vi "Tom_Bentham_Flux.vi"() -> (5 "Plug in titles":string[](array[string]), 7 "Plug in values":string[](array[string]))   [LabVIEW 2010]
uses:
  Globals/Plug_in_data_global.vi
  Globals/Meas_global.vi
  Globals/LDA_meas_global_1.vi
panel:
  in  "FFID  Channel":u16(ring)=2 items=["LDA (U)", "LDA (W)", "FF (C) Sync", "FF (C)"]
  in  "Flux velocity Channel":u16(ring) items=["LDA (U)", "LDA (W)", "FF (C) Sync", "FF (C)"]
  out "Flux":cluster{"Histogram of X":dbl[], "Axis":dbl[]}(graph)
  out "FF":cluster{"Histogram of X":dbl[], "Axis":dbl[]}(graph)
  out "LDA 1st Comp":cluster{"Histogram of X":dbl[], "Axis":dbl[]}(graph)
  out "LDA 2nd Comp":cluster{"Histogram of X":dbl[], "Axis":dbl[]}(graph)
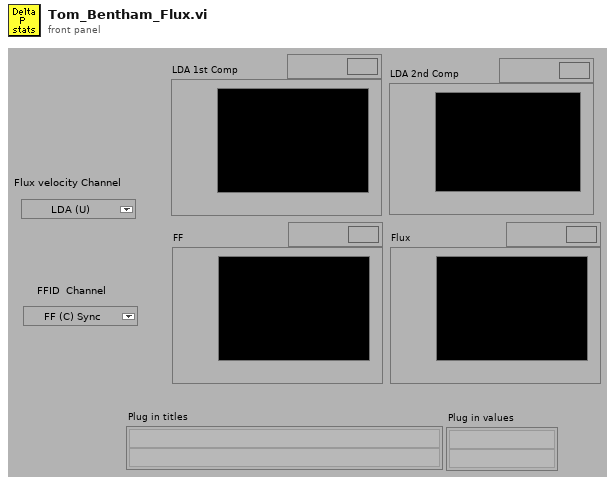
[diagram p1: front panel]
types:
  T1 = typedef "Analysis_info_cluster.ctl" = cluster{"Colour":u32, "Inst type":T2, "Inst name":string, "Symbol":string, "Code name":string, "Extra Info":string, "Inst Array":T3, "Index":i32, "Voltage Index":i32, "Extra Titles":string[], "Extra Values":string[]}
  T2 = typedef "Inst_type.ctl" = enum16{"Propeller anemometer", "Raw voltage", "Pressure Transducer", "Pitot-static tube", "Preston tube", "Hot wire", "Cross wire 1", "Cross wire 2", "Generic Linear", "Generic Polynomial", "Generic BackPoly", "Fast FID", "Thermocouple", "Cold wire", "Pulsed Wire", "LDA Vel", "LDA Tran time", "LDA Arr time"}
  T3 = typedef "Instrument_Array.ctl" = enum16{"PWA", "LDA", "Analogue"}
  T4 = enum16{"Save no data", "Save data in new files", "Save data in existing files"}
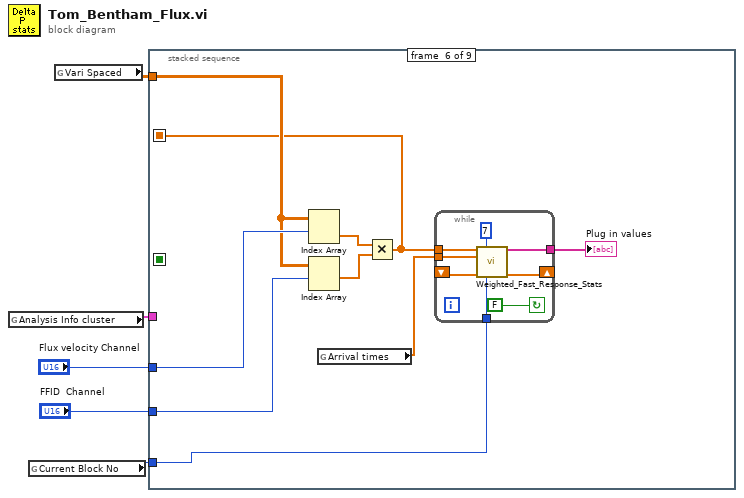
[diagram p0: block diagram]
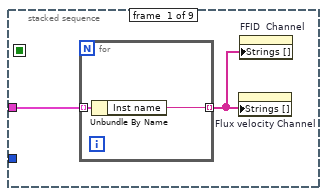
[diagram p2: hidden frame]
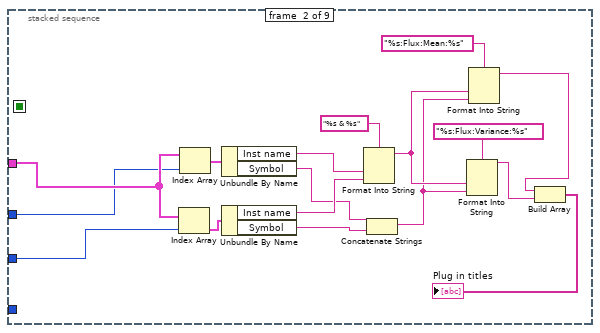
[diagram p3: hidden frame]
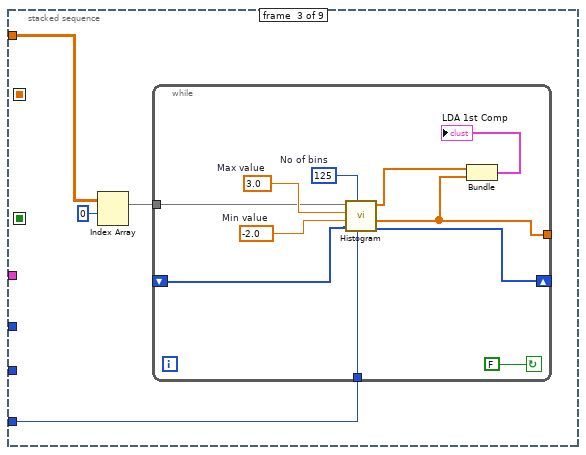
[diagram p4: hidden frame]
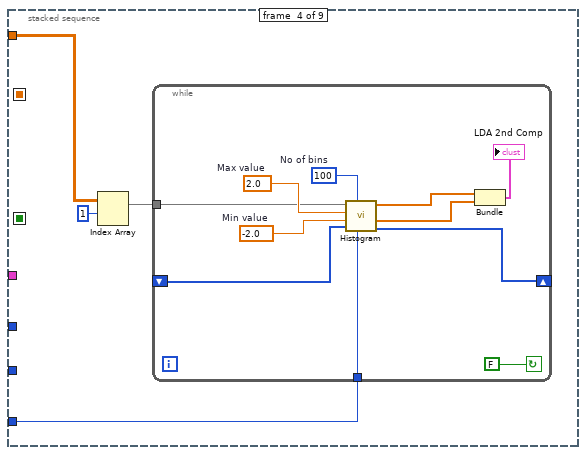
[diagram p5: hidden frame]
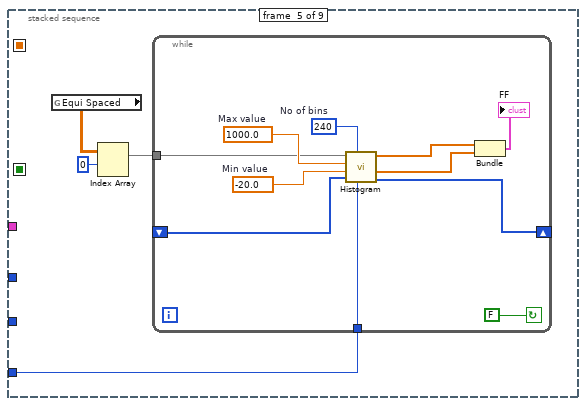
[diagram p6: hidden frame]
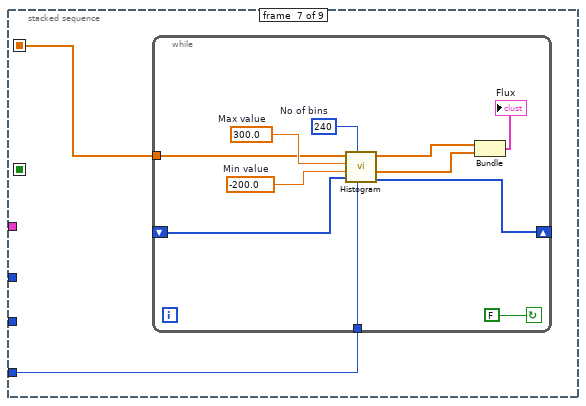
[diagram p7: hidden frame]
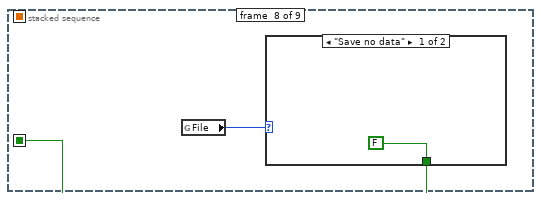
[diagram p8: hidden frame]
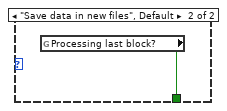
[diagram p9: hidden frame]
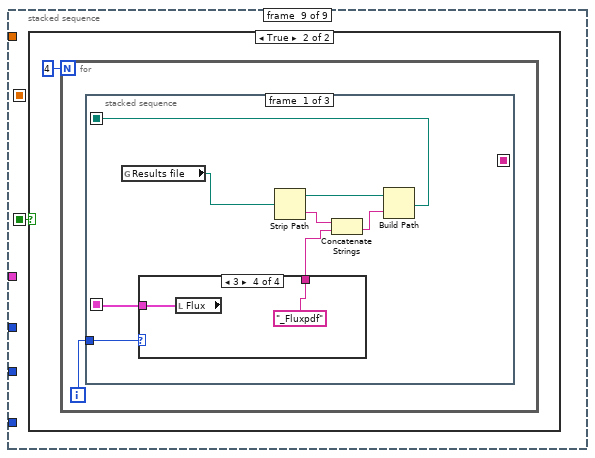
[diagram p10: hidden frame]
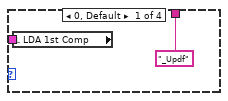
[diagram p12: hidden frame]
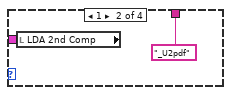
[diagram p13: hidden frame]
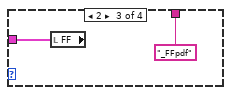
[diagram p14: hidden frame]
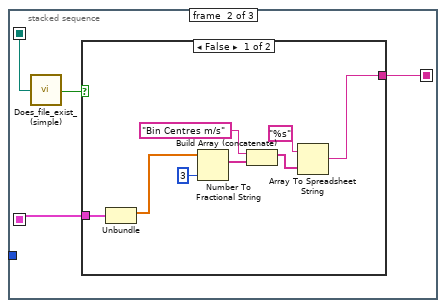
[diagram p15: hidden frame]
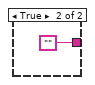
[diagram p16: hidden frame]
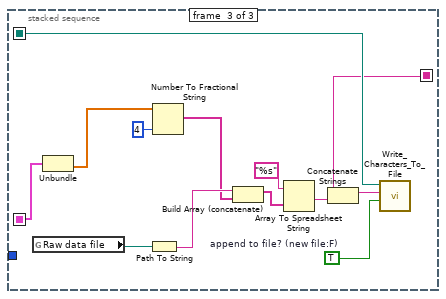
[diagram p17: hidden frame]
diagram:
  n1 = global read "Meas_global.vi" "Analysis Info cluster"() -> (w3:T1[])
  n2 = global read "Meas_global.vi" "Current Block No"() -> (w4:i32)
  n3 = global read "Plug_in_data_global.vi" "Vari Spaced"() -> (w5:dbl[][])
  n4 = stacked-sequence {
    seq-local: [_ _ _ _ _ w72 _ _ _] -> [_ _ _ _ _ _ w89 _ _]
    seq-local: [_ _ _ _ _ _ _ w102 _] -> [_ _ _ _ _ _ _ _ w106]
    tunnel: w5 -> [_ _ w28 w43 _ w79 _ _ _]
    tunnel: w4 -> [_ _ w30 w45 w60 w73 w90 _ _]
    tunnel: w3 -> [w7 w26 _ _ _ _ _ _ _]
    tunnel: "Flux velocity Channel" -> [_ w11 _ _ _ w80 _ _ _]
    tunnel: "FFID  Channel" -> [_ w10 _ _ _ w78 _ _ _]
    frame #0 {
      n5 = for {
        tunnel: w7 -> [w9] mode=indexing
        tunnel: [w8] -> w6 mode=indexing
        n6 = Unbundle By Name(w9) -> ("Inst name"=w8:string)
      }
      n7 = property on="Flux velocity Channel" class="Ring (strict)"("Strings []"=w6) -> ()  [unwired: 2 in, 2 out]
      n8 = property on="FFID  Channel" class="Ring (strict)"("Strings []"=w6) -> ()  [unwired: 2 in, 2 out]
    }
    frame #1 {
      n9 = Index Array(array=w26, index=w10) -> (element=w24:T1)
      n10 = Index Array(array=w26, index=w11) -> (element=w25:T1)
      n11 = Unbundle By Name(w25) -> ("Inst name"=w22:string, "Symbol"=w20:string)
      n12 = Unbundle By Name(w24) -> ("Inst name"=w23:string, "Symbol"=w19:string)
      n13 = Format Into String(format string="%s & %s" ("Format String"), w22, w23) -> (resulting string=w16:string)  [unwired: 2 in, 1 out]
      n14 = Concatenate Strings(w20, w19) -> (w15:string)
      n15 = Format Into String(format string="%s:Flux:Variance:%s" ("Format String"), w16, w15) -> (resulting string=w13:string)  [unwired: 2 in, 1 out]
      n16 = Format Into String(format string="%s:Flux:Mean:%s" ("Format String"), w16, w15) -> (resulting string=w14:string)  [unwired: 2 in, 1 out]
      n17 = Build Array(w14, w13) -> (→"Plug in titles":string[])
    }
    frame #2 {
      n18 = Index Array(array=w28, index (row)=0) -> (element=w27:dbl[])  [unwired: 1 in]
      n19 = while {
        tunnel: w27 -> [w35]
        tunnel: w30 -> [w37]
        tunnel: [w33] -> _
        shift-left: _ -> [w36]
        shift-right: [w40] -> _
        stop <- FALSE continue-if-true
        w38 = 3.0  # Max value
        w39 = -2.0  # Min value
        w41 = 125  # No of bins
        n20 = call "Histogram.vi"("Current Block No"=w37, "No of bins"=w41, "Shift Hist"=w36, "Min value"=w39, "Max value"=w38, "X"=w35) -> ("Shift Hist"=w40:i32[], "Histogram of X"=w33:dbl[], "Axis"=w34:dbl[])  [unwired: 1 in, 1 out]
        n21 = Bundle("Axis"=w34, "Histogram of X"=w33) -> (→"LDA 1st Comp":cluster{"Axis":dbl[], "Histogram of X":dbl[]})  [unwired: 1 out]
      }
    }
    frame #3 {
      n22 = Index Array(array=w43, index (row)=1) -> (element=w42:dbl[])  [unwired: 1 in]
      n23 = while {
        tunnel: w42 -> [w50]
        tunnel: w45 -> [w52]
        shift-left: _ -> [w51]
        shift-right: [w55] -> _
        stop <- FALSE continue-if-true
        w53 = 2.0  # Max value
        w54 = -2.0  # Min value
        w56 = 100  # No of bins
        n24 = call "Histogram.vi"("Current Block No"=w52, "No of bins"=w56, "Shift Hist"=w51, "Min value"=w54, "Max value"=w53, "X"=w50) -> ("Shift Hist"=w55:i32[], "Histogram of X"=w47:dbl[], "Axis"=w48:dbl[])  [unwired: 1 in, 1 out]
        n25 = Bundle("Axis"=w48, "Histogram of X"=w47) -> (→"LDA 2nd Comp":cluster{"Axis":dbl[], "Histogram of X":dbl[]})  [unwired: 1 out]
      }
    }
    frame #4 {
      n26 = global read "Plug_in_data_global.vi" "Equi Spaced"() -> (w57:dbl[][])
      n27 = Index Array(array=w57, index (row)=0) -> (element=w58:dbl[])  [unwired: 1 in]
      n28 = while {
        tunnel: w58 -> [w65]
        tunnel: w60 -> [w67]
        shift-left: _ -> [w66]
        shift-right: [w70] -> _
        stop <- FALSE continue-if-true
        w68 = 1000.0  # Max value
        w69 = -20.0  # Min value
        w71 = 240  # No of bins
        n29 = call "Histogram.vi"("Current Block No"=w67, "No of bins"=w71, "Shift Hist"=w66, "Min value"=w69, "Max value"=w68, "X"=w65) -> ("Shift Hist"=w70:i32[], "Histogram of X"=w63:dbl[], "Axis"=w64:dbl[])  [unwired: 1 in, 1 out]
        n30 = Bundle("Axis"=w64, "Histogram of X"=w63) -> (→"FF":cluster{"Axis":dbl[], "Histogram of X":dbl[]})  [unwired: 1 out]
      }
    }
    frame #5 {
      n31 = Index Array(array=w79, index (row)=w80) -> (element=w77:dbl[])  [unwired: 1 in]
      n32 = Index Array(array=w79, index (row)=w78) -> (element=w76:dbl[])  [unwired: 1 in]
      n33 = global read "LDA_meas_global_1.vi" "Arrival times"() -> (w75:dbl[])
      n34 = Multiply(x=w77, y=w76) -> (x*y=w72:dbl[])
      n35 = while {
        tunnel: w73 -> [w82]
        tunnel: [w83] -> w74
        tunnel: w75 -> [w85]
        tunnel: w72 -> [w86]
        shift-left: _ -> [w88]
        shift-right: [w87] -> _
        stop <- FALSE continue-if-true
        n36 = call "Weighted_Fast_Response_Stats.vi"("U"=w86, "Index"=7, "Weighting"=w85, "Shift in"=w88, "Block No"=w82) -> ("Results file string array"=w83:string[], "Shift out"=w87:dbl[])  [unwired: 1 in, 8 out]
      }
      "Plug in values" <- w74
    }
    frame #6 {
      n37 = while {
        tunnel: w89 -> [w95]
        tunnel: w90 -> [w97]
        shift-left: _ -> [w96]
        shift-right: [w100] -> _
        stop <- FALSE continue-if-true
        w98 = 300.0  # Max value
        w99 = -200.0  # Min value
        w101 = 240  # No of bins
        n38 = call "Histogram.vi"("Current Block No"=w97, "No of bins"=w101, "Shift Hist"=w96, "Min value"=w99, "Max value"=w98, "X"=w95) -> ("Shift Hist"=w100:i32[], "Histogram of X"=w93:dbl[], "Axis"=w94:dbl[])  [unwired: 1 in, 1 out]
        n39 = Bundle("Axis"=w94, "Histogram of X"=w93) -> (→"Flux":cluster{"Axis":dbl[], "Histogram of X":dbl[]})  [unwired: 1 out]
      }
    }
    frame #7 {
      n40 = global read "Meas_global.vi" "File"() -> (w103:T4)
      n41 = case shown="\"Save no data\"" w103 {
        tunnel: [FALSE w105] -> w102
        frame "Save no data" {
        }
        frame "Save data in new files", Default {
          n42 = global read "Meas_global.vi" "Processing last block?"() -> (w105:bool)
        }
      }
    }
    frame #8 {
      n43 = case shown="True" w106 {
        frame False {
        }
        frame True {
          n44 = for {
            N: 4 -> [_]
            i -> [w108]
            n45 = stacked-sequence {
              seq-local: [w111 _ _] -> [_ w126 w143]
              seq-local: [w110 _ _] -> [_ w128 w142]
              seq-local: [_ w125 _] -> [_ _ w139]
              tunnel: w108 -> [w113 _ _]
              frame #0 {
                n46 = global read "Meas_global.vi" "Results file"() -> (w109:path)
                n47 = case shown="3" w113 {
                  tunnel: ["_Updf" ("Substring") "_U2pdf" ("Substring") "_FFpdf" ("Substring") "_Fluxpdf" ("Substring")] -> w112
                  tunnel: [w117 w119 w121 w123] -> w111
                  frame 0, Default {
                    n48 = local read "LDA 1st Comp"() -> (w117:cluster{"Histogram of X":dbl[], "Axis":dbl[]})
                  }
                  frame 1 {
                    n49 = local read "LDA 2nd Comp"() -> (w119:cluster{"Histogram of X":dbl[], "Axis":dbl[]})
                  }
                  frame 2 {
                    n50 = local read "FF"() -> (w121:cluster{"Histogram of X":dbl[], "Axis":dbl[]})
                  }
                  frame 3 {
                    n51 = local read "Flux"() -> (w123:cluster{"Histogram of X":dbl[], "Axis":dbl[]})
                  }
                }
                n52 = Strip Path(path=w109) -> (stripped path=w116:path, name=w115:string)
                n53 = Concatenate Strings(w115, w112) -> (w114:string)
                n54 = Build Path(base path=w116, name or relative path=w114) -> (appended path=w110:path)
              }
              frame #1 {
                n55 = call "Does_file_exist_(simple).vi"("Pathname"=w128) -> ("exists?"=w127:bool)
                n56 = case shown="False" w127 {
                  tunnel: w126 -> [w136 _]
                  tunnel: [w129 ""] -> w125
                  frame False {
                    n57 = Unbundle(w136) -> ("Histogram of X"=w134:dbl[])  [unwired: 1 out]
                    n58 = Number To Fractional String(number=w134, precision (6)=i16 3) -> (F-format string=w131:string[])  [unwired: 2 out]
                    n59 = Build Array (concatenate)("Bin Centres m/s" ("Input Element"), w131) -> (w133:string[])
                    n60 = Array To Spreadsheet String(array=w133, 3:"%s" ("format string")) -> (spreadsheet string=w129:string)  [unwired: 1 out]
                  }
                  frame True {
                  }
                }
              }
              frame #2 {
                w144 = TRUE  # append to file? (new file:F)
                n61 = global read "Meas_global.vi" "Raw data file"() -> (w149:path)
                n62 = Unbundle(w143) -> ("Axis"=w141:dbl[])  [unwired: 1 out]
                n63 = Path To String(path=w149) -> (string=w148:string)
                n64 = Number To Fractional String(number=w141, precision (6)=i16 4) -> (F-format string=w147:string[])  [unwired: 2 out]
                n65 = Build Array (concatenate)(w148, w147) -> (w146:string[])
                n66 = Array To Spreadsheet String(array=w146, 3:"%s" ("format string")) -> (spreadsheet string=w140:string)  [unwired: 1 out]
                n67 = Concatenate Strings(w139, w140) -> (w138:string)
                n68 = call "Write_Characters_To_File.vi"("file path (dialog if empty)"=w142, "character string"=w138, "append to file? (new file:F)"=w144) -> ()  [unwired: 2 in, 4 out]
              }
            }
          }
        }
      }
    }
  }
